vi "RM-save-command.vi"(8 "错误输入（无错误）":errorcluster, 11 "MB_Master_Serial输入":refnum<class "MB_Master_Serial.lvclass">) -> (0 "错误输出":errorcluster, 3 "MB_Master_Serial输出":refnum<class "MB_Master_Serial.lvclass">)   [LabVIEW 2014]
uses:
  <vilib>/Plasmionique/MB Master/MB_Master_Serial/MB_Master_Serial.lvclass
  <vilib>/Plasmionique/MB Master/MB Master.lvlib
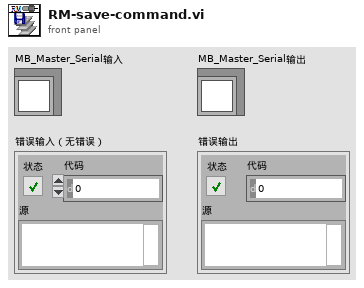
[diagram p1: front panel]
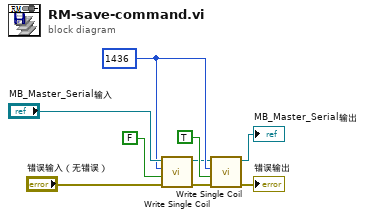
[diagram p0: block diagram]
diagram:
  w5 = u16 1436 ("address")
  n1 = call <vilib>:"Write Single Coil.vi"("error in (no error)"="错误输入（无错误）", "value"=FALSE, "address"=w5, "MB session in"="MB_Master_Serial输入") -> ("error out"=w2:errorcluster, "MB session out"=w3:refnum<class "MB_Master_Serial.lvclass">)  [unwired: 6 in]
  n2 = call <vilib>:"Write Single Coil.vi"("error in (no error)"=w2, "value"=TRUE, "address"=w5, "MB session in"=w3) -> ("error out"=→"错误输出":errorcluster, "MB session out"=→"MB_Master_Serial输出":refnum<class "MB_Master_Serial.lvclass">)  [unwired: 6 in]
